vi "Configure DO Manual.vi"(0 "VISA resource name":refnum<visa-resource-name>, 5 "Channel Number (0001)":string="0001", 7 "Span And Energize":T1={"Span Lower Limit (0)"=0, "Span Upper Limit (1)"=1, "Unit (\"\")"="", "Output (De-Energize) "=FALSE} {"Span Upper Limit (1)" min=1 max=32; "Span Lower Limit (0)" min=1 max=32}, 11 "error in (no error)":errorcluster) -> (4 "VISA resource name out":refnum<visa-resource-name>, 6 "Channel Number":string, 15 "error out":errorcluster)   [LabVIEW 2020, in "Yokogawa GX Series.lvlib"]
doc: "Sets the DO manual output related settings.\n\nCommand: SRangeDO"
uses:
  <instrlib>/Yokogawa GX Series/Yokogawa GX Series.lvlib
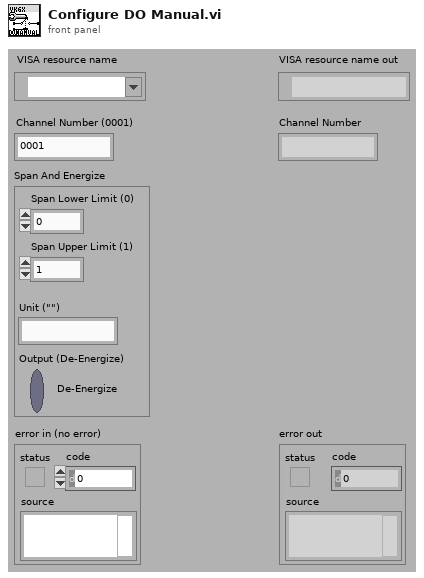
[diagram p1: front panel]
types:
  T1 = cluster{"Span Lower Limit (0)":i32, "Span Upper Limit (1)":i32, "Unit (\"\")":string, "Output (De-Energize) ":bool}
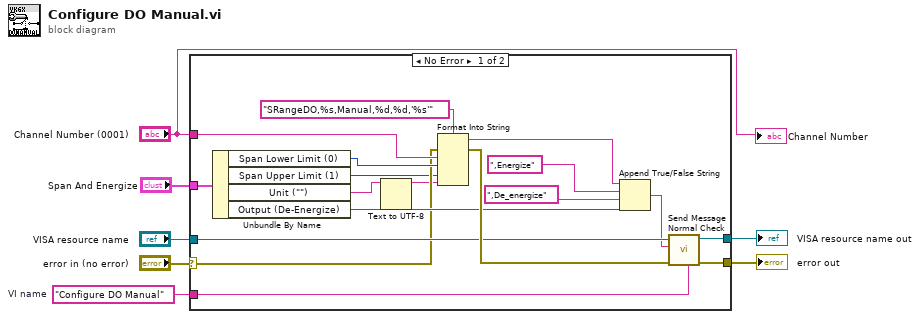
[diagram p0: block diagram]
diagram:
  w7 = "Configure DO Manual"  # VI name
  n1 = case shown="No Error" "error in (no error)" {
    selector: "error in (no error)" -> [w11 w26]
    tunnel: w7 -> [w25 _]
    tunnel: [w24 w27] -> w6
    tunnel: [w23 w26] -> w5
    tunnel: "VISA resource name" -> [w17 w27]
    tunnel: "Span And Energize" -> [w16 _]
    tunnel: "Channel Number (0001)" -> [w12 _]
    frame No Error {
      n2 = Unbundle By Name(w16) -> ("Span Lower Limit (0)"=w15:i32, "Span Upper Limit (1)"=w10:i32, "Unit (\"\")"=w9:string, "Output (De-Energize)"=w14:bool)
      n3 = Text to UTF-8(11:w9) -> (3:w8:string)  [unwired: 2 in, 1 out]
      n4 = Format Into String(format string="SRangeDO,%s,Manual,%d,%d,'%s'" ("形式文字列"), error in=w11, w12, w15, w10, w8) -> (resulting string=w19:string, error out=w18:errorcluster)  [unwired: 1 in]
      n5 = Append True/False String(1:w14, 2:",De_energize", 3:",Energize", 4:w19) -> (0:w13:string)
      n6 = call <instrlib>:"Send Message Normal Check.vi"("Source (\"\")"=w25, "error in (no error)"=w18, "Send Message (\"\")"=w13, "VISA resource name"=w17) -> ("error out"=w23:errorcluster, "VISA resource name out"=w24:refnum<visa-resource-name>)  [unwired: 1 in, 5 out]
    }
    frame Error {
    }
  }
  "error out" <- w5
  "VISA resource name out" <- w6
  "Channel Number" <- "Channel Number (0001)"
